vi "Data.Engine.Close.vi"(8 "error in":errorcluster, 11 "Plugin Data Access in":refnum<class "Plugin Data Access.lvclass">) -> (0 "error out":errorcluster, 3 "Plugin Data Access out":refnum<class "Plugin Data Access.lvclass">)   [LabVIEW 2024, in "VS Plugin Inline Async API.lvlib" / "Plugin Data Access.lvclass"]
uses:
  Plugin Data Access.lvclass
  Plugin Data Access.lvclass/Plugin Data Access.ctl
  Read/Read.lvclass
  Write/Write.lvclass
  ReadWrite/ReadWrite.lvclass
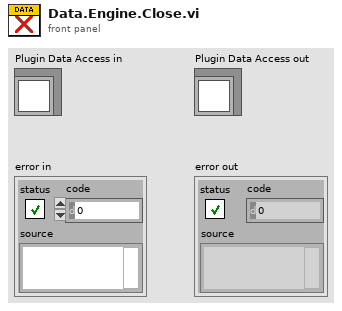
[diagram p1: front panel]
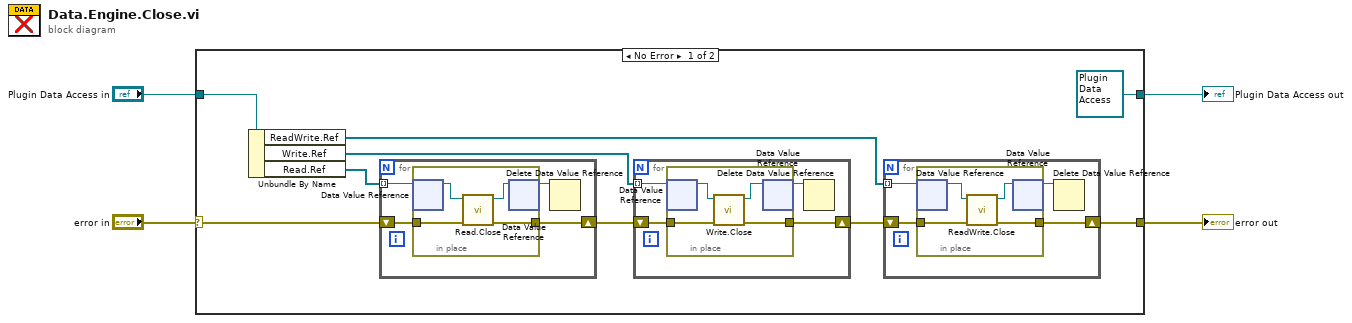
[diagram p0: block diagram]
diagram:
  n1 = case shown="No Error" "error in" {
    selector: "error in" -> [w13 w39]
    tunnel: [w11 w39] -> w3
    tunnel: [refnum<class "Plugin Data Access.lvclass"> refnum ("Data Access API in") w38] -> w1
    tunnel: "Plugin Data Access in" -> [w8 w38]
    frame No Error {
      n2 = Unbundle By Name(w8) -> ("ReadWrite.Ref"=w5:refnum<data-value>[], "Write.Ref"=w6:refnum<data-value>[], "Read.Ref"=w9:refnum<data-value>[])
      n3 = for {
        tunnel: w9 -> [w31] mode=indexing
        shift-right: [w32] -> w10
        shift-left: w13 -> [w33]
        n4 = in-place {
          in-place-border: w33 -> [w37]
          in-place-border: [w36] -> w32
          n5 = in-place-dvr #1(w31) -> (w35:refnum<class "Read.lvclass">)  [unwired: 1 out]
          n6 = call "Read.Close.vi"("error in"=w37, "Read in"=w35) -> ("error out"=w36:errorcluster, "Read out"=w34:refnum<class "Read.lvclass">)  [unwired: 8 in]
          n7 = in-place-dvr #1(w34) -> (w30:refnum<data-value>)  [unwired: 1 out]
        }
        n8 = Delete Data Value Reference(data value reference=w30) -> ()  [unwired: 1 in, 2 out]
      }
      n9 = for {
        tunnel: w6 -> [w23] mode=indexing
        shift-right: [w24] -> w12
        shift-left: w10 -> [w25]
        n10 = in-place {
          in-place-border: w25 -> [w29]
          in-place-border: [w28] -> w24
          n11 = in-place-dvr #2(w23) -> (w27:refnum<class "Write.lvclass">)  [unwired: 1 out]
          n12 = call "Write.Close.vi"("error in"=w29, "Write in"=w27) -> ("error out"=w28:errorcluster, "Write out"=w26:refnum<class "Write.lvclass">)  [unwired: 8 in]
          n13 = in-place-dvr #2(w26) -> (w22:refnum<data-value>)  [unwired: 1 out]
        }
        n14 = Delete Data Value Reference(data value reference=w22) -> ()  [unwired: 1 in, 2 out]
      }
      n15 = for {
        tunnel: w5 -> [w15] mode=indexing
        shift-right: [w16] -> w11
        shift-left: w12 -> [w17]
        n16 = in-place {
          in-place-border: w17 -> [w21]
          in-place-border: [w20] -> w16
          n17 = in-place-dvr #3(w15) -> (w19:refnum<class "ReadWrite.lvclass">)  [unwired: 1 out]
          n18 = call "ReadWrite.Close.vi"("error in"=w21, "ReadWrite in"=w19) -> ("error out"=w20:errorcluster, "ReadWrite out"=w18:refnum<class "ReadWrite.lvclass">)  [unwired: 8 in]
          n19 = in-place-dvr #3(w18) -> (w14:refnum<data-value>)  [unwired: 1 out]
        }
        n20 = Delete Data Value Reference(data value reference=w14) -> ()  [unwired: 1 in, 2 out]
      }
    }
    frame Error {
    }
  }
  "error out" <- w3
  "Plugin Data Access out" <- w1
